vi "Destroy.vi"(0 "reference in":refnum<class "Registration.lvclass">, 5 "error in (no error)":errorcluster) -> (14 "reference out":refnum<class "Registration.lvclass">, 19 "error out":errorcluster)   [LabVIEW 2020, in "Registration.lvclass"]
doc: "Destructor."
uses:
  Registration.lvclass
  Generic Utilities_class/Generic Utilities.lvclass
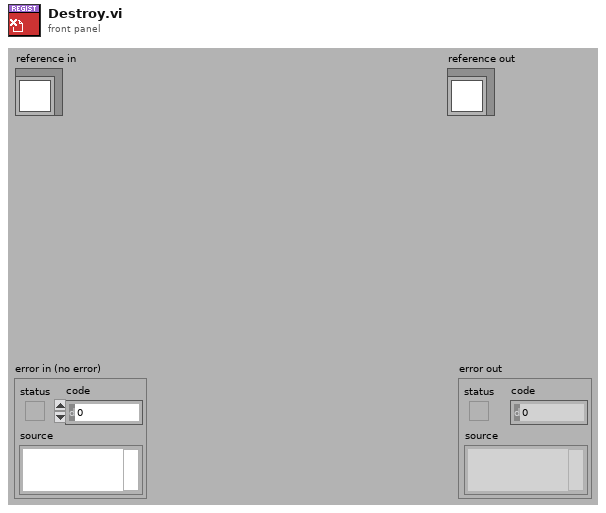
[diagram p1: front panel]
types:
  T1 = typedef "Registration.lvclass/ObjectAttributes.ctl" = cluster{"Registration Info":T2, "Object Origin":enum16{"New/Created", "Existing"}}
  T2 = typedef "Registration.lvclass/Registration Info.ctl" = cluster{"First Name":string, "Last Name":string, "Registration Code":string, "Registration Level":T3}
  T3 = typedef "Registration.lvclass/Registration Type.ctl" = enum16{"Unregistered", "Registered - Full Activation", "Not Required- Full Activation"}
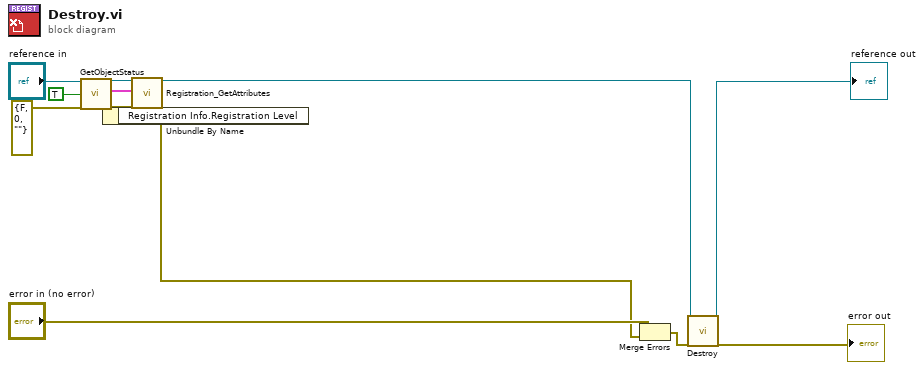
[diagram p0: block diagram]
diagram:
  n1 = call-dynamic "GetObjectStatus.vi"("reference in"="reference in", "simple info (F)"=TRUE ("simple info"), "error in (no error)"=errorcluster {"status"=FALSE, "code"=0, "source"=""}) -> ("reference out"=w5:refnum<class "Registration.lvclass">, "error out"=w6:errorcluster)  [unwired: 5 in, 10 out]
  n2 = call "Registration_GetAttributes.vi"("reference in"=w5, "error in (no error)"=w6) -> ("reference out"=w4:refnum<class "Registration.lvclass">, "attributes"=w3:T1, "error out"=w7:errorcluster)  [unwired: 14 in, 1 out]
  n3 = Unbundle By Name(w3) -> ()  [unwired: 1 out]
  n4 = Merge Errors("error in (no error)", w7) -> (w11:errorcluster)
  n5 = call-parent "Destroy.vi"("reference in"=w4, "error in (no error)"=w11) -> ("reference out"=→"reference out":refnum<class "Registration.lvclass">, "error out"=→"error out":errorcluster)  [unwired: 16 in]
